vi "Initialize.vi"(7 "ChannelName":string="Setpoint.ch%d.SP", 8 "error in":errorcluster, 9 "Number of Channels":u32=1, 10 "Instance Name":string, 11 "Overload Counter Channels in":refnum<class "Overload Counter Channels.lvclass">) -> (0 "error out":errorcluster, 3 "Overload Counter Channels out":refnum<class "Overload Counter Channels.lvclass">)   [LabVIEW 2023, in "Overload Counter Channels.lvclass"]
uses:
  Overload Counter Channels.lvclass
  Overload Counter Channels.lvclass/Overload Counter Channels.ctl
  <vilib>/ADAS Replay HIL/Channels/Tag Wrapper/Polymorphic/Open Producer Tag (Double).vi
  <vilib>/ADAS Replay HIL/Channels/Tag Wrapper/Polymorphic/Set Default Value (Double).vi
  <vilib>/ADAS Replay HIL/Channels/Tag Wrapper/Polymorphic/Open Producer Tag (Double).vi/45cd6eaa-a1ce-41a4-8aba-62a49d103d7e.vi
  <vilib>/ADAS Replay HIL/Channels/Tag Wrapper/Polymorphic/Set Default Value (Double).vi/228e99de-6fcf-414d-86fc-dc277c7b351f.vi
  <vilib>/ADAS Replay HIL/Channels/Tag Wrapper/Polymorphic/Open Producer Tag (Double).vi/45cd6eaa-a1ce-41a4-8aba-62a49d103d7e.vi/c28b0ead-42ad-4072-80a2-aca7f2bd7ce3.vi
  <vilib>/ADAS Replay HIL/Channels/Tag Wrapper/Polymorphic/Set Default Value (Double).vi/228e99de-6fcf-414d-86fc-dc277c7b351f.vi/4bc1c15b-36ab-481f-b8dd-c64075ce723a.vi
  <vilib>/ADAS Replay HIL/AdasHilServices/AdasHilServices Fill In Error Info Ex.vi
  Utilities/Utilities.lvlib
  <vilib>/ADAS Replay HIL/Channels/Tag Wrapper/Tag Wrapper.lvlib
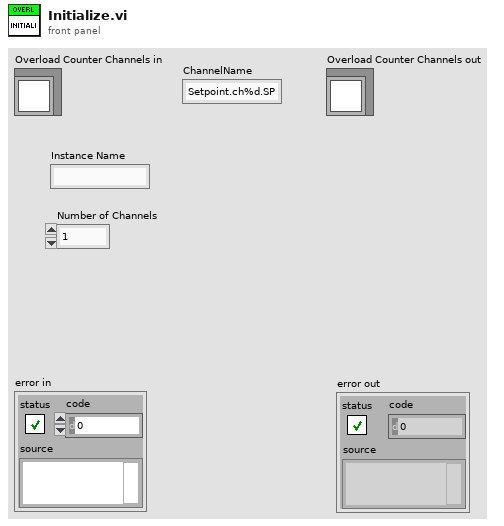
[diagram p1: front panel]
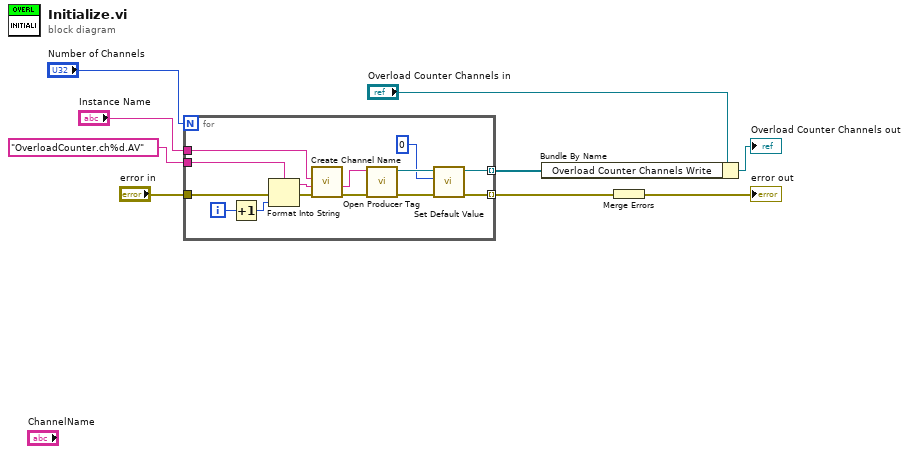
[diagram p0: block diagram]
diagram:
  n1 = for {
    N: "Number of Channels" -> [_]
    tunnel: "Instance Name" -> [w15]
    tunnel: "error in" -> [w11]
    tunnel: [w20] -> w3 mode=indexing
    tunnel: "OverloadCounter.ch%d.AV" ("ChannelName") -> [w16]
    tunnel: [w13] -> w4 mode=indexing
    i -> [w17]
    n2 = Increment(x=w17) -> (x+1=w18:i32)
    n3 = Format Into String(format string=w16, error in=w11, w18) -> (resulting string=w14:string, error out=w12:errorcluster)  [unwired: 1 in]
    n4 = call "Create Channel Name.vi"("error in"=w12, "Channel Name"=w14, "Plugin Name"=w15) -> ("error out"=w22:errorcluster, "Data Channel Name"=w19:string)  [unwired: 7 in]
    n5 = call-poly <vilib>:"Open Producer Tag.vi"("error in"=w22, "Channel Name"=w19) -> ("error out"=w21:errorcluster, "ADAS HIL Channel"=w23:refnum<k21>)  [unwired: 8 in]
    n6 = call-poly <vilib>:"Set Default Value.vi"("error in"=w21, "Default Value"=0, "ADAS HIL Channel in"=w23) -> ("error out"=w20:errorcluster, "ADAS HIL Channel out"=w13:refnum<k21>)  [unwired: 7 in]
  }
  n7 = Bundle By Name(cluster="Overload Counter Channels in", "Overload Counter Channels Write"=w4) -> (→"Overload Counter Channels out":refnum<class "Overload Counter Channels.lvclass">)
  n8 = Merge Errors(w3) -> (→"error out":errorcluster)
